vi "DT_Triangle Manager_Format.vi"(4 "p 3 triangle":i32, 6 "p 2 triangle":i32, 7 "CCW? [T]":bool=TRUE, 8 "p 1 triangle":i32, 9 "p 3":i32, 10 "p 2":i32, 11 "p 1":i32) -> (3 "Triangle":i32[](array[numeric]))   [LabVIEW 2017, in "NI_AAL_Geometry.lvlib"]
uses:
  <vilib>/Analysis/NI_AAL_Geometry.lvlib
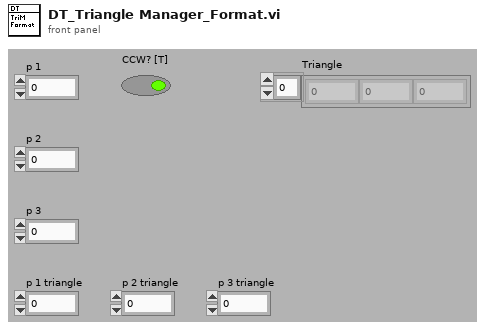
[diagram p1: front panel]
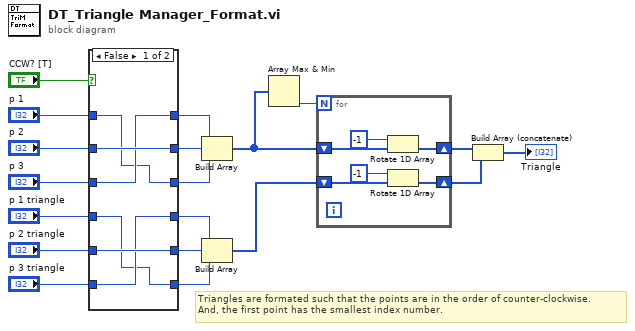
[diagram p0: block diagram]
diagram:
  # "Triangles are formated such that the points are in the order of counter-clockwise.\nAnd, the first point has the smallest index number."
  n1 = case shown="False" "CCW? [T]" {
    tunnel: "p 1" -> [w23 w31]
    tunnel: "p 3" -> [w24 w29]
    tunnel: "p 2" -> [w25 w30]
    tunnel: [w24 w31] -> w11
    tunnel: [w25 w30] -> w10
    tunnel: [w23 w29] -> w9
    tunnel: "p 1 triangle" -> [w20 w28]
    tunnel: [w21 w28] -> w5
    tunnel: "p 3 triangle" -> [w21 w27]
    tunnel: [w20 w27] -> w2
    tunnel: "p 2 triangle" -> [w22 w26]
    tunnel: [w22 w26] -> w3
    frame False {
    }
    frame True {
    }
  }
  n2 = Build Array(w11, w10, w9) -> (w8:i32[])
  n3 = Build Array(w5, w3, w2) -> (w1:i32[])
  n4 = Array Max & Min(array=w8) -> (min index (indices)=w18:i32)  [unwired: 3 out]
  n5 = for {
    N: w18 -> [_]
    shift-right: [w35] -> w17
    shift-left: w8 -> [w37]
    shift-right: [w32] -> w15
    shift-left: w1 -> [w33]
    n6 = Rotate 1D Array(1:w37, 2:-1 ("n")) -> (0:w35:i32[])
    n7 = Rotate 1D Array(1:w33, 2:-1 ("n")) -> (0:w32:i32[])
  }
  n8 = Build Array (concatenate)(w17, w15) -> (→"Triangle":i32[])
